vi "Andon Get Shift.vi"(6 "CID":string[](array[string]), 8 "error in (no error)":errorcluster, 9 "Current Time":timestamp, 10 "Time Stamp Out":timestamp[](array[timestamp]), 11 "connection reference in":T1) -> (0 "error out":errorcluster, 2 "Shift":i32, 3 "connection reference out":T1)   [LabVIEW 2017]
uses:
  <vilib>/addons/database/Connection.llb/Conn ObjectReference.ctl
  1f78dfa2-1741-423b-aba4-8dcc2f8f7b67.vi
  <vilib>/addons/database/Connection.llb/Conn Execute.vi
  <vilib>/addons/database/Recordset.llb/Rec Fetch Recordset Data (R).vi
  <vilib>/addons/database/Recordset.llb/Rec Destroy - Connection.vi
  <vilib>/addons/database/_DB Variant To Data/Database Variant To Data.xnode
  <vilib>/addons/database/NI_Database_API.lvlib
  <userlib>/_OpenG.lib/comparison/comparison.llb/I32 Changed__ogtk.vi
panel:
  in  "Station Array":u32[](array[numeric])
  out "double precision float":dbl format="%#_13g"
  in  "Shift Time Details":T2 {"3End" format="%<%H:%M:%S\n%x>T"; "2End" format="%<%H:%M:%S\n%x>T"; "3Start" format="%<%H:%M:%S\n%x>T"; "2Start" format="%<%H:%M:%S\n%x>T"; "1End" format="%<%H:%M:%S\n%x>T"; "1Start" format="%<%H:%M:%S\n%x>T"}
  # "Start Time"
  # "End Time"
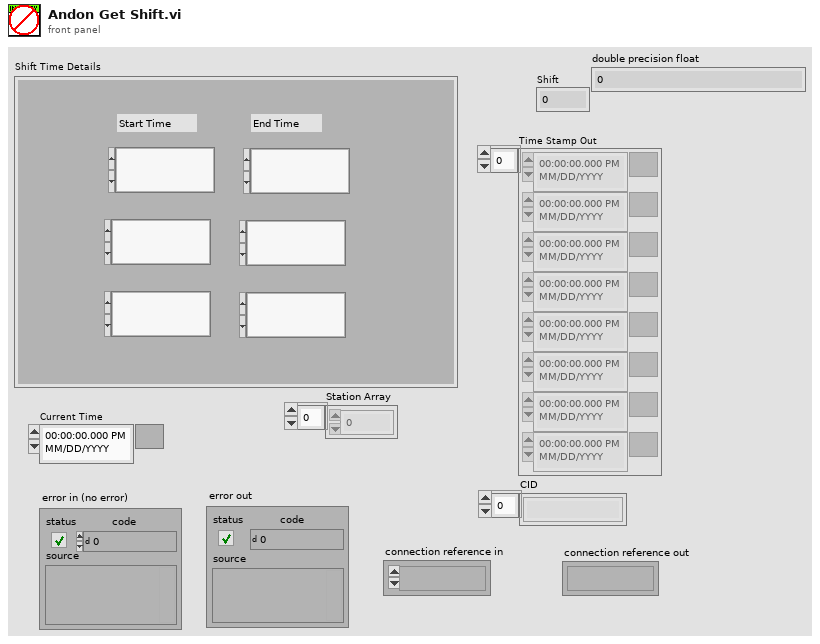
[diagram p1: front panel]
types:
  T1 = typedef "NI_Database_API.lvlib/Conn ObjectReference.ctl" = refnum<k1>
  T2 = cluster{"1Start":timestamp, "1End":timestamp, "2Start":timestamp, "3Start":timestamp, "2End":timestamp, "3End":timestamp}
  T3 = typedef "LVDateTimeRec.ctl" = cluster{"fractional second":dbl, "second":i32, "minute":i32, "hour":i32, "day of month":i32, "month":i32, "year":i32, "day of week":i32, "day of year":i32, "DST":i32}
  T4 = typedef "NI_Database_API.lvlib/Rec ObjectReference.ctl" = refnum<k1>
  T5 = cluster{i32, i32, i32, i32, "date/time string":string, "Date String":string}
  T6 = cluster{i32, "date/time string":string, i32, i32, i32, "Date String":string}
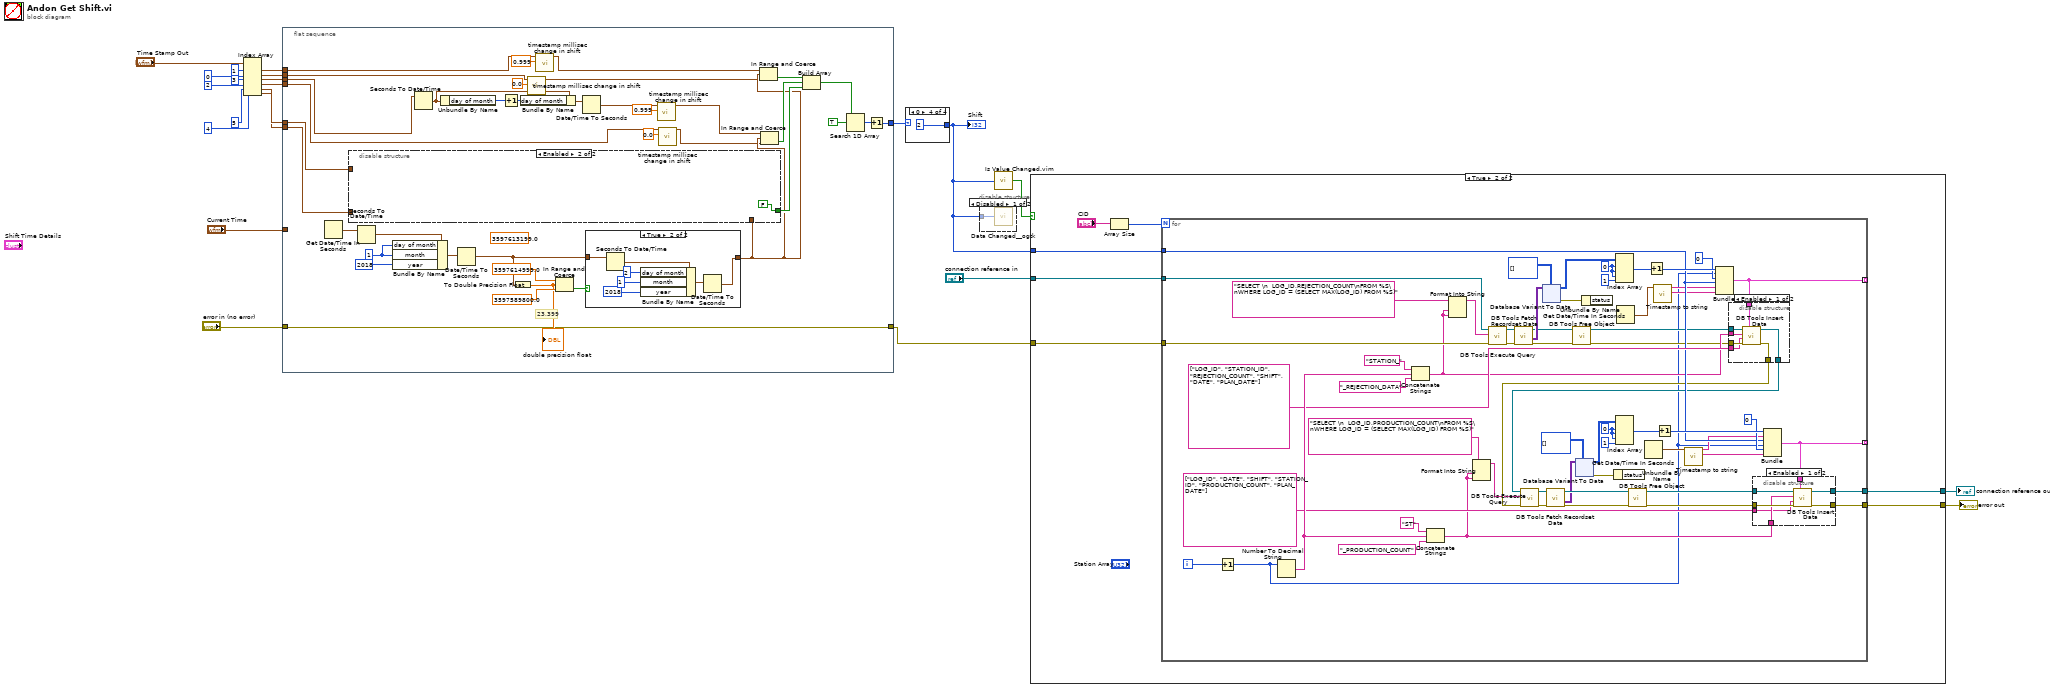
[diagram p0: block diagram]
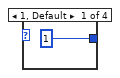
[diagram p6: hidden frame]
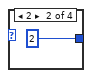
[diagram p7: hidden frame]
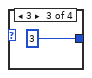
[diagram p8: hidden frame]
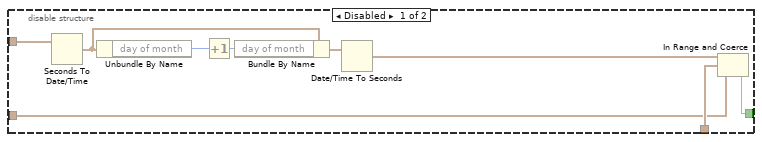
[diagram p9: hidden frame]
diagram:
  n1 = Index Array(array="Time Stamp Out", index #1=1 ("index"), index #2=0 ("index"), index #3=3 ("index"), index #4=2 ("index"), index #5=5 ("index"), index #6=4 ("index")) -> (element #1=w17:timestamp, element #2=w16:timestamp, element #3=w13:timestamp, element #4=w12:timestamp, element #5=w9:timestamp, element #6=w8:timestamp)
  n2 = flat-sequence {
    tunnel: [w54] -> w7
    tunnel: "error in (no error)" -> [w43]
    tunnel: [w43] -> w3
    tunnel: "Current Time" -> [_]
    tunnel: w17 -> [w34]
    tunnel: w16 -> [w30]
    tunnel: w13 -> [w35]
    tunnel: w12 -> [w25]
    tunnel: w9 -> [w42]
    tunnel: w8 -> [w41]
    frame #0 {
      (unwired) 3597613199.0 ("double precision float 2")
      w47 = 1 ("day of month")
      # "23,399"
      n3 = Get Date/Time In Seconds() -> (seconds since 1Jan1904=w40:timestamp)
      n4 = Seconds To Date/Time(time stamp (now)=w40) -> (date time rec=w51:T3)  [unwired: 1 in]
      n5 = Bundle By Name(cluster=w51, "day of month"=w47, "month"=w47, "year"=2018) -> (w53:T3)
      n6 = Seconds To Date/Time(time stamp (now)=w35) -> (date time rec=w38:T3)  [unwired: 1 in]
      n7 = Unbundle By Name(w38) -> ("day of month"=w36:i32)
      n8 = Date/Time To Seconds(2:w53) -> (0:w45:timestamp)  [unwired: 1 in]
      n9 = Increment(x=w36) -> (x+1=w37:i32)
      n10 = To Double Precision Float(number=w45) -> (double precision float=w48:dbl)
      "double precision float" <- w48
      n11 = Bundle By Name(cluster=w38, "day of month"=w37) -> (w39:T3)
      n12 = call "timestamp millisec change in shift.vi"("fractional second"=0.0, "time stamp in"=w30) -> ("time stamp out"=w29:timestamp)  [unwired: 9 in]
      n13 = call "timestamp millisec change in shift.vi"("fractional second"=0.999, "time stamp in"=w34) -> ("time stamp out"=w33:timestamp)  [unwired: 9 in]
      n14 = In Range and Coerce(upper limit=3597614999.0 ("double precision float 2"), x=w48, lower limit=3597589800.0 ("double precision float")) -> (In Range?=w46:bool)  [unwired: 1 out]
      n15 = Date/Time To Seconds(2:w39) -> (0:w28:timestamp)  [unwired: 1 in]
      n16 = case shown="True" w46 {
        tunnel: w45 -> [w71 w74]
        tunnel: [w71 w73] -> w44
        frame False {
        }
        frame True {
          n17 = Seconds To Date/Time(time stamp (now)=w74) -> (date time rec=w76:T3)  [unwired: 1 in]
          n18 = Bundle By Name(cluster=w76, "day of month"=2, "month"=1 ("day of month"), "year"=2018) -> (w78:T3)
          n19 = Date/Time To Seconds(2:w78) -> (0:w73:timestamp)  [unwired: 1 in]
        }
      }
      n20 = disable-structure shown="Enabled" {
        disable-tunnel: [w68 FALSE] -> w58
        disable-tunnel: w44 -> [w67 _]
        disable-tunnel: w42 -> [w66 _]
        disable-tunnel: w41 -> [w65 _]
        frame Disabled {
          n21 = Seconds To Date/Time(time stamp (now)=w66) -> (date time rec=w63:T3)  [unwired: 1 in]
          n22 = Unbundle By Name(w63) -> ("day of month"=w61:i32)
          n23 = Increment(x=w61) -> (x+1=w62:i32)
          n24 = Bundle By Name(cluster=w63, "day of month"=w62) -> (w64:T3)
          n25 = Date/Time To Seconds(2:w64) -> (0:w69:timestamp)  [unwired: 1 in]
          n26 = In Range and Coerce(upper limit=w69, x=w67, lower limit=w65) -> (In Range?=w68:bool)  [unwired: 1 out]
        }
        frame Enabled {
        }
      }
      n27 = call "timestamp millisec change in shift.vi"("fractional second"=0.999, "time stamp in"=w28) -> ("time stamp out"=w27:timestamp)  [unwired: 9 in]
      n28 = call "timestamp millisec change in shift.vi"("fractional second"=0.0, "time stamp in"=w25) -> ("time stamp out"=w24:timestamp)  [unwired: 9 in]
      n29 = In Range and Coerce(upper limit=w33, x=w44, lower limit=w29) -> (In Range?=w60:bool)  [unwired: 1 out]
      n30 = In Range and Coerce(upper limit=w27, x=w44, lower limit=w24) -> (In Range?=w59:bool)  [unwired: 1 out]
      n31 = Build Array(w60, w59, w58) -> (w57:bool[])
      n32 = Search 1D Array(1D array=w57, element=TRUE) -> (index of element=w55:i32)  [unwired: 1 in]
      n33 = Increment(x=w55) -> (x+1=w54:i32)
    }
  }
  n34 = case shown="0" w7 {
    tunnel: [1 2 3 2] -> w2
    frame 1, Default {
    }
    frame 2 {
    }
    frame 3 {
    }
    frame 0 {
    }
  }
  "Shift" <- w2
  n35 = disable-structure shown="Disabled" {
    disable-tunnel: w2 -> [w83 _]
    frame Disabled {
      n36 = call-poly <userlib>:"Data Changed__ogtk.vi"("I32"=w83) -> ()  [unwired: 1 out]
    }
    frame Enabled {
    }
  }
  n37 = call "Is Value Changed.vim"("value"=w2) -> ("changed or first call?"=w1:bool)
  n38 = case shown="True" w1 {
    tunnel: [w85 w92] -> w6
    tunnel: "connection reference in" -> [w85 w91]
    tunnel: w2 -> [_ w90]
    tunnel: [w84 w89] -> w4
    tunnel: w3 -> [w84 w88]
    frame False {
    }
    frame True {
      n39 = Array Size(array="CID") -> (size(s)=w86:i32)
      n40 = for {
        N: w86 -> [_]
        tunnel: [w135] -> w89
        tunnel: [w134] -> w92
        tunnel: w91 -> [w128]
        tunnel: w90 -> [w133]
        tunnel: w88 -> [w127]
        tunnel: [w106] -> _ mode=indexing
        tunnel: [w105] -> _ mode=indexing
        i -> [w94]
        w144 = 0 ("index (row)")
        w147 = 0 ("index (row)")
        n41 = Increment(x=w94) -> (x+1=w93:i32)
        n42 = Number To Decimal String(number=w93) -> (decimal integer string=w141:string)  [unwired: 1 in]
        n43 = Concatenate Strings("STATION_" ("String"), w141, "_REJECTION_DATA" ("string")) -> (w122:string)
        n44 = Concatenate Strings("ST" ("String"), w141, "_PRODUCTION_COUNT" ("string")) -> (w107:string)
        n45 = Format Into String(format string="SELECT \n  LOG_ID,REJECTION_COUNT\nFROM %S\nWHERE LOG_ID = (SELECT MAX(LOG_ID) FROM %S)" ("SQL query"), w122, w122) -> (resulting string=w125:string)  [unwired: 2 in, 1 out]
        n46 = Format Into String(format string="SELECT \n  LOG_ID,PRODUCTION_COUNT\nFROM %S\nWHERE LOG_ID = (SELECT MAX(LOG_ID) FROM %S)" ("SQL query"), w107, w107) -> (resulting string=w108:string)  [unwired: 2 in, 1 out]
        n47 = call-poly <vilib>:"DB Tools Execute Query.vi"("error in (no error)"=w127, "SQL query"=w125, "connection reference"=w128) -> ("error out"=w132:errorcluster, "recordset reference"=w103:T4)  [unwired: 5 in]
        n48 = call-poly <vilib>:"DB Tools Fetch Recordset Data.vi"("error in (no error)"=w132, "recordset reference"=w103) -> ("error out"=w129:errorcluster, "recordset data"=w131:variant[][], "recordset reference out"=w104:T4)  [unwired: 3 in]
        n49 = xnode "Database Variant To Data"("database variant"=w131, "type"=i32[][] []) -> ("data"=w124:i32[][], "error out"=w123:errorcluster)  [unwired: 1 in]
        n50 = call-poly <vilib>:"DB Tools Free Object.vi"("error in (no error)"=w129, "recordset reference"=w104) -> ("error out"=w102:errorcluster, "connection reference"=w101:T1)  [unwired: 8 in]
        n51 = Unbundle By Name(w123) -> ()  [unwired: 1 out]
        n52 = Index Array(array=w124, index (row) #1=w147, index (col) #1=w147, index (row) #2=w147, index (col) #2=1 ("disabled index (col)")) -> (element #1=w151:i32)  [unwired: 1 out]
        n53 = Get Date/Time In Seconds() -> (seconds since 1Jan1904=w100:timestamp)
        n54 = Get Date/Time In Seconds() -> (seconds since 1Jan1904=w99:timestamp)
        n55 = Increment(x=w151) -> (x+1=w152:i32)
        n56 = call "Timestamp to string.vi"("time stamp"=w100) -> ("Date String"=w95:string, "date/time string"=w96:string)  [unwired: 8 in, 1 out]
        n57 = call "Timestamp to string.vi"("time stamp"=w99) -> ("Date String"=w97:string, "date/time string"=w98:string)  [unwired: 8 in, 1 out]
        n58 = Bundle(w152, w93, 0, w133, "date/time string"=w96, "Date String"=w95) -> (w105:T5)  [unwired: 1 in]
        n59 = disable-structure shown="Enabled" {
          disable-tunnel: w122 -> [w256 _]
          disable-tunnel: w101 -> [w255 w258]
          disable-tunnel: w102 -> [w254 w257]
          disable-tunnel: w105 -> [w253 _]
          disable-tunnel: string[] ["LOG_ID", "STATION_ID", "REJECTION_COUNT", "SHIFT", "DATE", "PLAN_DATE"] ("columns") -> [w252 _]
          disable-tunnel: [w251 w258] -> w115
          disable-tunnel: [w250 w257] -> w114
          frame Enabled {
            n60 = call <vilib>:"DB Tools Insert Data.vi"("data"=w253, "error in (no error)"=w254, "columns"=w252, "table"=w256, "connection reference"=w255) -> ("error out"=w250:errorcluster, "connection reference out"=w251:T1)  [unwired: 5 in]
          }
          frame Disabled {
          }
        }
        n61 = call-poly <vilib>:"DB Tools Execute Query.vi"("error in (no error)"=w114, "SQL query"=w108, "connection reference"=w115) -> ("error out"=w119:errorcluster, "recordset reference"=w118:T4)  [unwired: 5 in]
        n62 = call-poly <vilib>:"DB Tools Fetch Recordset Data.vi"("error in (no error)"=w119, "recordset reference"=w118) -> ("error out"=w121:errorcluster, "recordset data"=w110:variant[][], "recordset reference out"=w120:T4)  [unwired: 3 in]
        n63 = xnode "Database Variant To Data"("database variant"=w110, "type"=i32[][] []) -> ("data"=w111:i32[][], "error out"=w113:errorcluster)  [unwired: 1 in]
        n64 = Unbundle By Name(w113) -> ()  [unwired: 1 out]
        n65 = Index Array(array=w111, index (row) #1=w144, index (col) #1=w144, index (row) #2=w144, index (col) #2=1 ("disabled index (col)")) -> (element #1=w136:i32)  [unwired: 1 out]
        n66 = call-poly <vilib>:"DB Tools Free Object.vi"("error in (no error)"=w121, "recordset reference"=w120) -> ("error out"=w117:errorcluster, "connection reference"=w116:T1)  [unwired: 8 in]
        n67 = Increment(x=w136) -> (x+1=w138:i32)
        n68 = Bundle(w138, "date/time string"=w98, w133, w93, 0, "Date String"=w97) -> (w106:T6)  [unwired: 1 in]
        n69 = disable-structure shown="Enabled" {
          disable-tunnel: w117 -> [w247 w248]
          disable-tunnel: w116 -> [w246 w249]
          disable-tunnel: w107 -> [w245 _]
          disable-tunnel: string[] ["LOG_ID", "DATE", "SHIFT", "STATION_ID", "PRODUCTION_COUNT", "PLAN_DATE"] ("columns") -> [w244 _]
          disable-tunnel: w106 -> [w243 _]
          disable-tunnel: [w242 w248] -> w135
          disable-tunnel: [w241 w249] -> w134
          frame Enabled {
            n70 = call <vilib>:"DB Tools Insert Data.vi"("data"=w243, "error in (no error)"=w247, "columns"=w244, "table"=w245, "connection reference"=w246) -> ("error out"=w242:errorcluster, "connection reference out"=w241:T1)  [unwired: 5 in]
          }
          frame Disabled {
          }
        }
      }
    }
  }
  "error out" <- w4
  "connection reference out" <- w6
